vi "CommonVIs_ClassIconSelection.vi"(3 "Offset":T1, 4 "SaveChangesInClassRightAway(True)":bool=TRUE, 5 "IconSelected":refnum<user-event>, 6 "IconsToShow(All)":T2, 7 "Icon":refnum<vi>, 8 "error in (no error)":errorcluster, 9 "Messages(Stop or Empty string will stop this VI)":refnum<user-event>, 10 "IconSelection":refnum<vi>, 11 "LVClassToActOn":refnum<vi>) -> ()   [LabVIEW 2020]
uses:
  <resource>/Framework/Providers/Open_GDS/ClassProviders/Common/CommonVIs/CommonVIs_ClassIconSelection_Action.ctl
  <vilib>/Utility/miscctls.llb/LVPositionTypeDef.ctl
  45c64d35-ac36-4efc-be44-fe8a67d8f3b0.vi
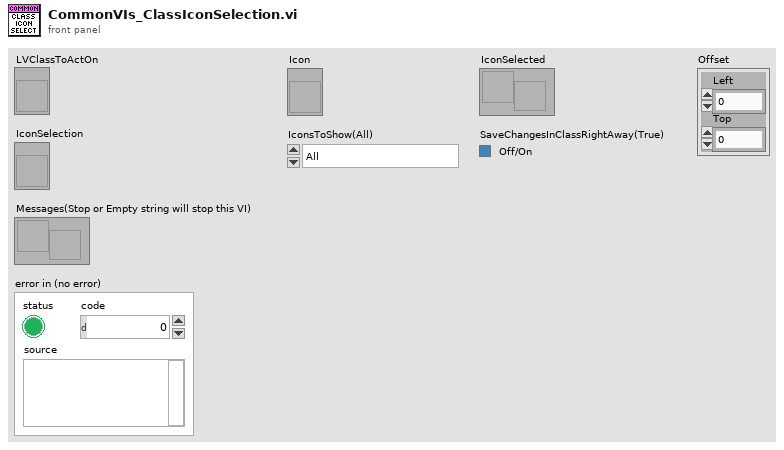
[diagram p1: front panel]
types:
  T1 = typedef "LVPositionTypeDef.ctl" = cluster{"Left":i32, "Top":i32}
  T2 = typedef "CommonVIs_ClassIconSelection_Action.ctl" = enum16{"All", "Non Interface", "Only Interface"}
  T3 = cluster{"SelectedIcon":string, "IconSelection":picture, "CurrentIcon":picture, "Icons":string[][], "MarkedIconSelection":picture, "Timeout":i32}
  T4 = cluster{"Width":i16, "Style":enum32{"Solid", "Dash", "Dot", "DashDot", "DashDotDot"}}
  T5 = cluster{"left":i16, "top":i16, "right":i16, "bottom":i16}
  T6 = typedef "BaseProvider_IniFileSettings.ctl" = cluster{"ClassFolderSuffix":string, "InterfaceFolderSuffix":string, "InterfaceIcon":string}
  T7 = typedef "imagedata.ctl" = cluster{"image type":i32, "image depth":i32, "image":u8[], "mask":u8[], "colors":u32[], "Rectangle":cluster{"left":i16, "top":i16, "right":i16, "bottom":i16}}
  T8 = cluster{"index of element":i32, i32, "index of element":i32, i32}
  T9 = cluster{"IconDimensions":i16, "IconDimensions":i16, "IconDimensions":i16, "IconDimensions":i16}
  T10 = cluster{"index of element":i16, i16, "index of element":i16, i16}
  T11 = typedef "lveventtype.ctl" = enum32{"Null", "Timeout", "Annotation Menu Selection", "Annotation Menu Selection?", "App Instance Close", "App Instance Close?", "Autoscale Range Change", "Bookmark Info Change", "Cell Edit", "Cell Edit?", "Cursor Grab", "Cursor Grab?", "Cursor Menu Selection", "Cursor Menu Selection?", "Cursor Move", "Cursor Release", "Data Change", "Direction Change", "Display State Change", "Drag Ended", "Drag Enter", "Drag Leave", "Drag Over", "Drag Source Update", "Drag Starting", "Drag Starting?", "Drop", "Exec State Change", "Key Down", "Key Down?", "Key Repeat", "Key Repeat?", "Key Up", "Listbox Double Click", "Menu Activation?", "Menu Selection (App)", "Menu Selection? (App)", "Menu Selection (User)", "Mouse Down", "Mouse Down?", "Mouse Enter", "Mouse Leave", "Mouse Move", "Mouse Up", "Mouse Wheel", "NI Security User Change (App)", "Pane Size", "Panel Close", "Panel Close?", "Panel Resize", "Plot Attribute Change", "Scale Range Change", "Shortcut Menu Activation?", "Shortcut Menu Selection (App)", "Shortcut Menu Selection? (App)", "Shortcut Menu Selection (User)", "Tree Double Click", "Tree Drag", "Tree Drag?", "Tree Drop", "Tree Drop?", "Tree Item Close", "Tree Item Close?", "Tree Item Open", "Tree Item Open?", "User Event", "Value Change"}
  T12 = typedef "LVMouseTypeDef.ctl" = cluster{"Mouse Position":cluster{"X":i32, "Y":i32}, "Mouse Modifiers":cluster{"Button Down":bool, "Shift Mod":bool, "Menu Mod":bool, "Option Mod":bool}}
  T13 = cluster{"IconDimensions":i16, "IconDimensions":i16}
  T14 = typedef "Scripting_ConnectorPanePatternType.ctl" = u16
  T15 = typedef "GOOP_WireConfigurationType.ctl" = cluster{"Edge thickness":i32, "Edge color":u32, "Center thickness":i32, "Center pattern":T16, "CenterColor1":u32, "CenterColor2":u32, "Tunnels and terminals colors":u32}
  T16 = typedef "GOOP_WirePattern.ctl" = enum16{"Solid", "Large dash", "Small dash"}
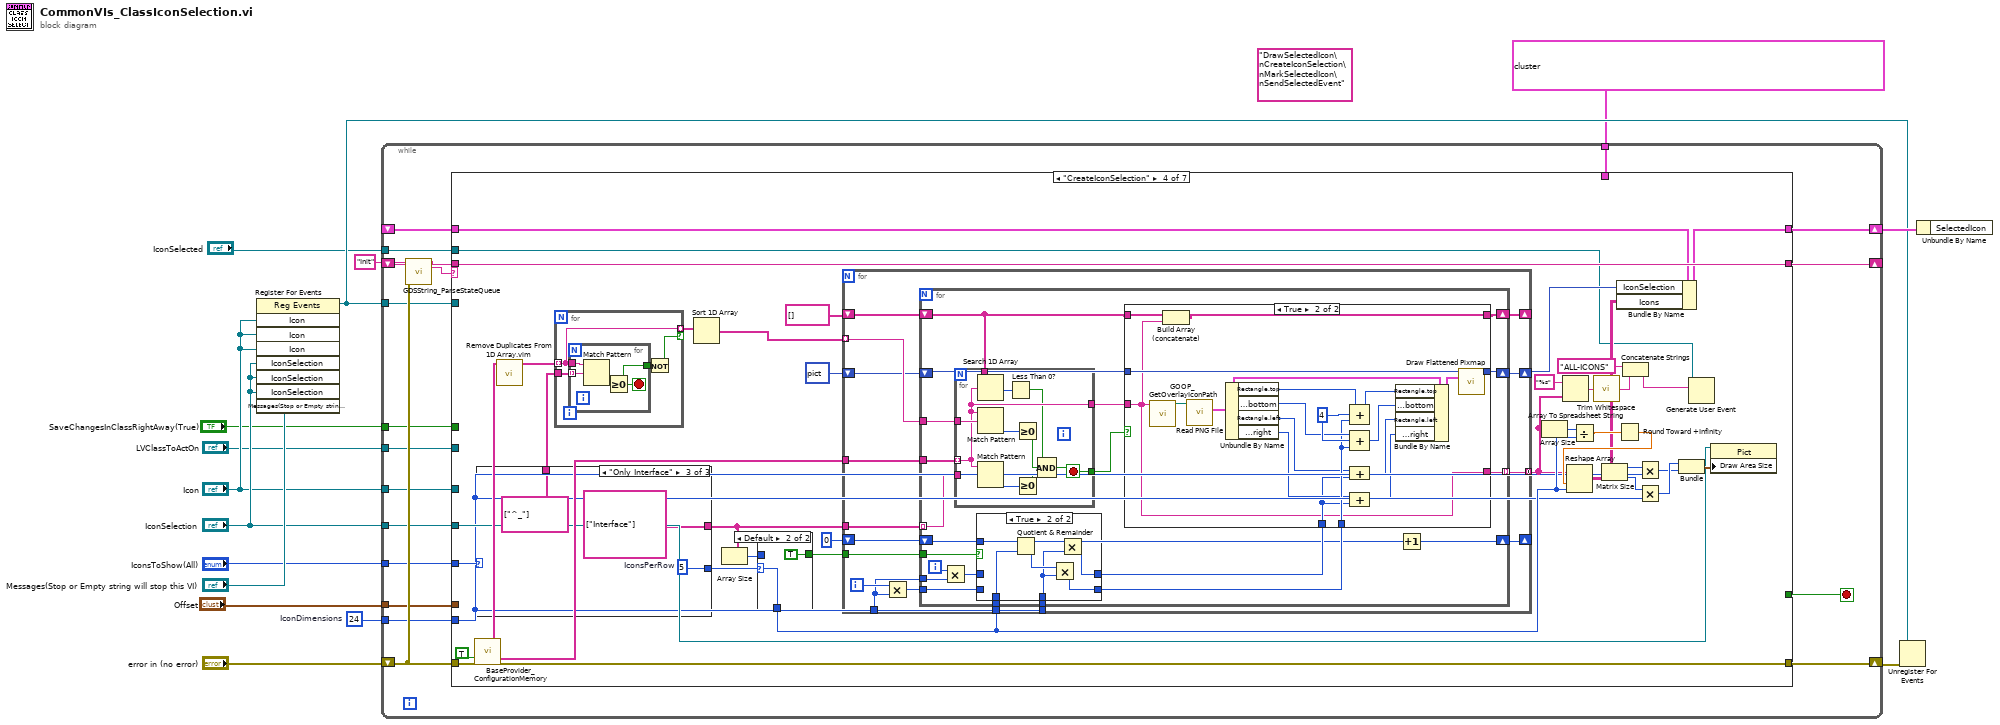
[diagram p0: block diagram]
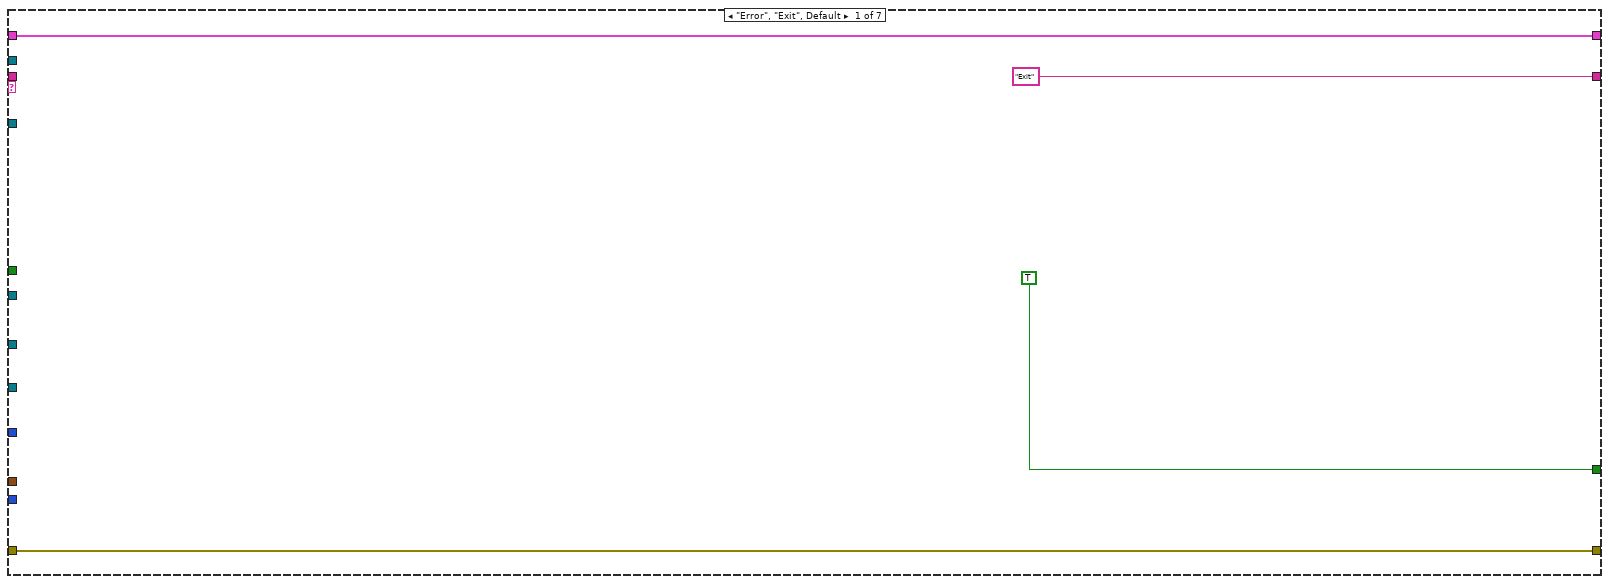
[diagram p2: hidden frame]
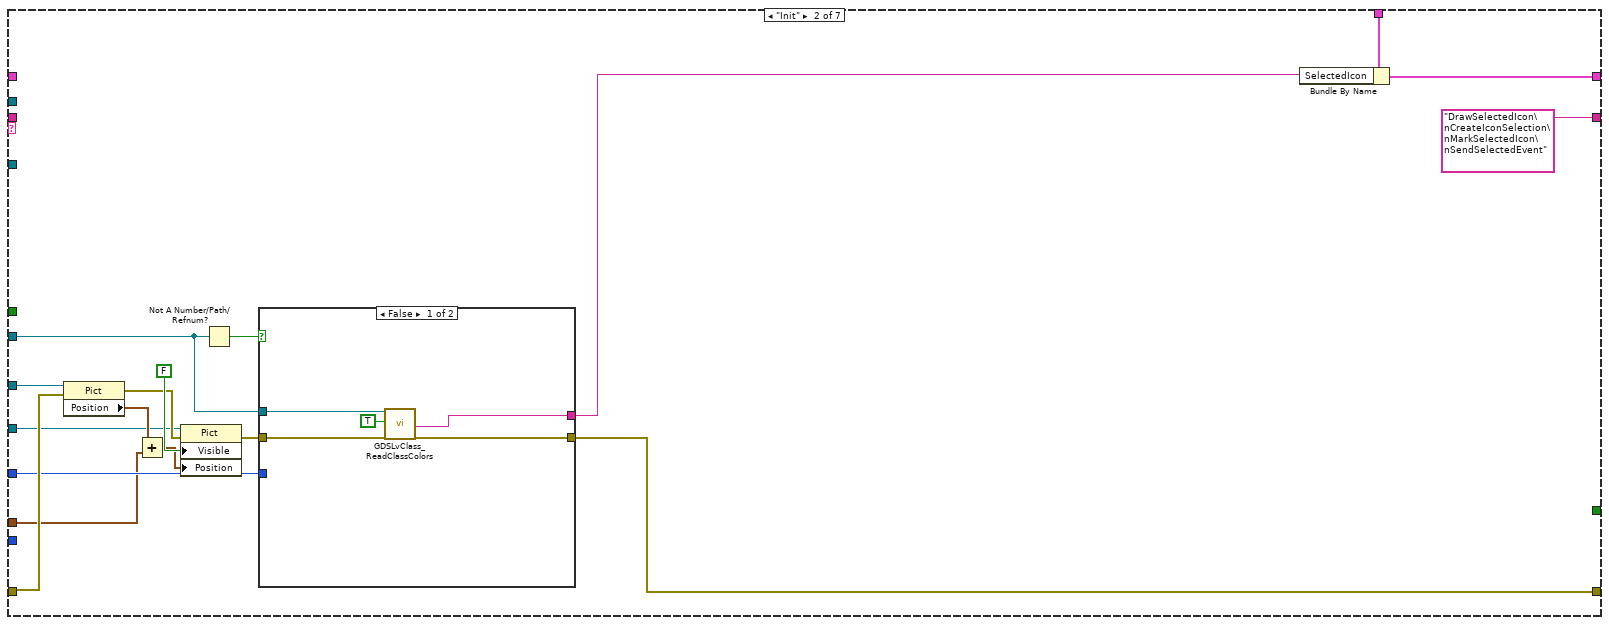
[diagram p3: hidden frame]
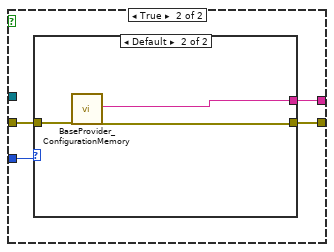
[diagram p4: hidden frame]
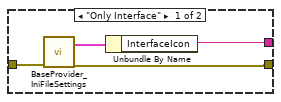
[diagram p5: hidden frame]
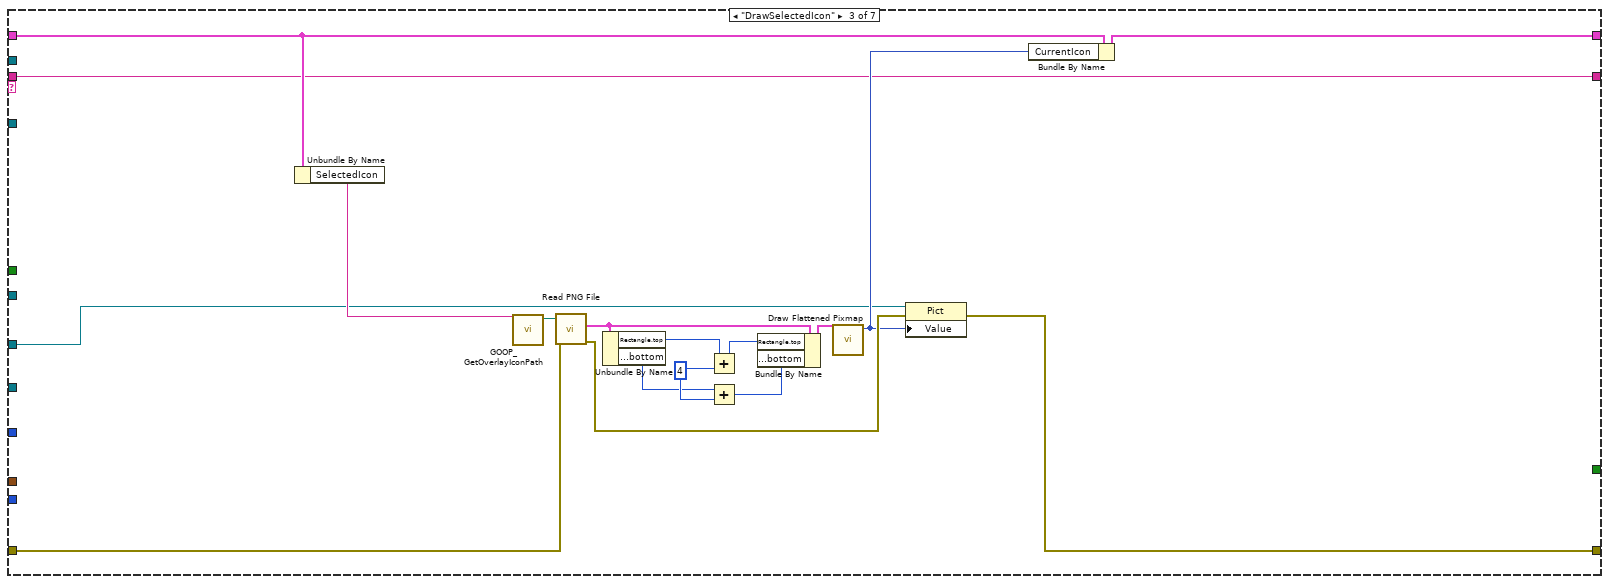
[diagram p6: hidden frame]
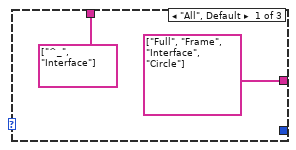
[diagram p8: hidden frame]
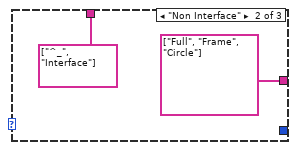
[diagram p9: hidden frame]
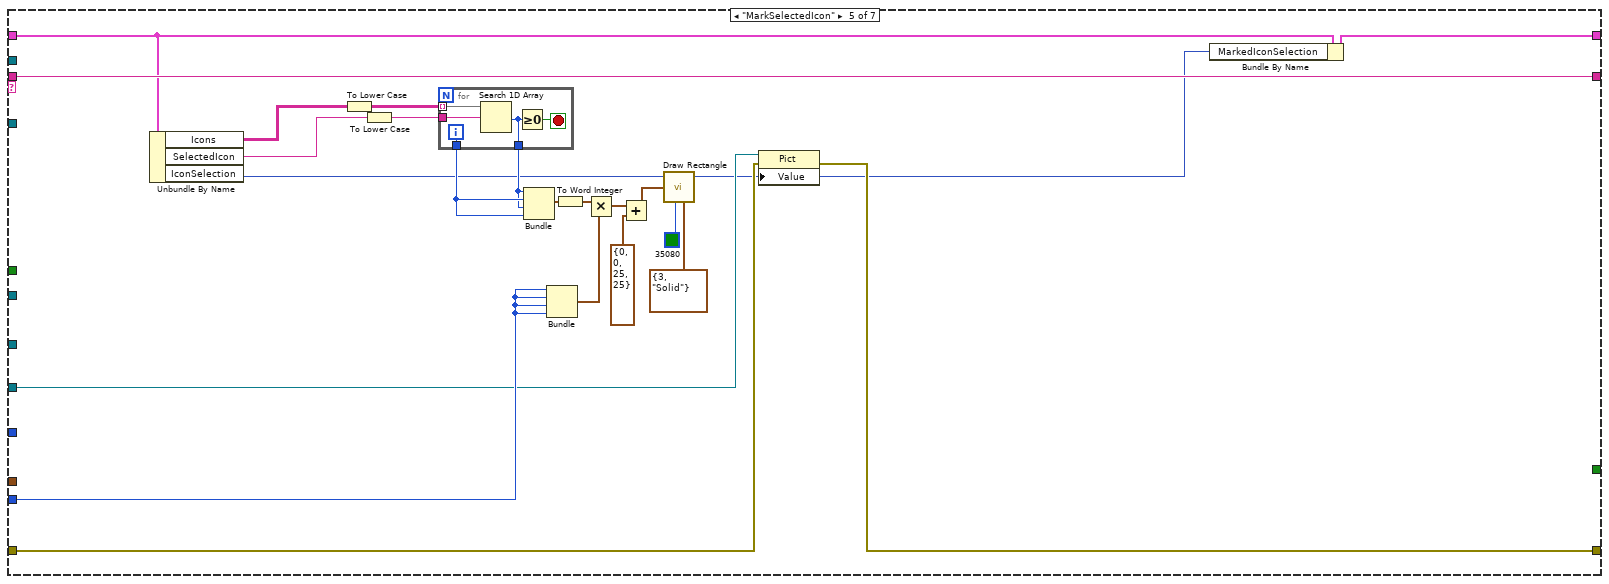
[diagram p12: hidden frame]
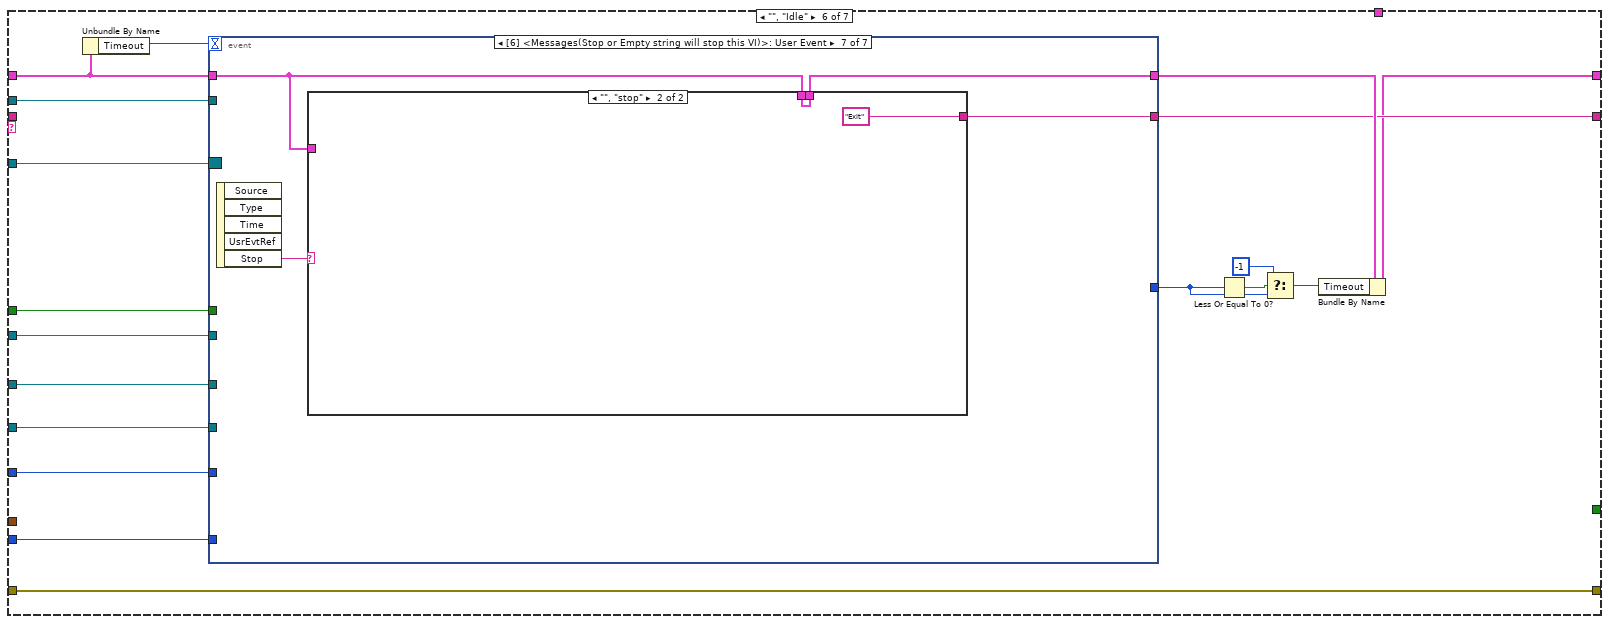
[diagram p13: hidden frame]
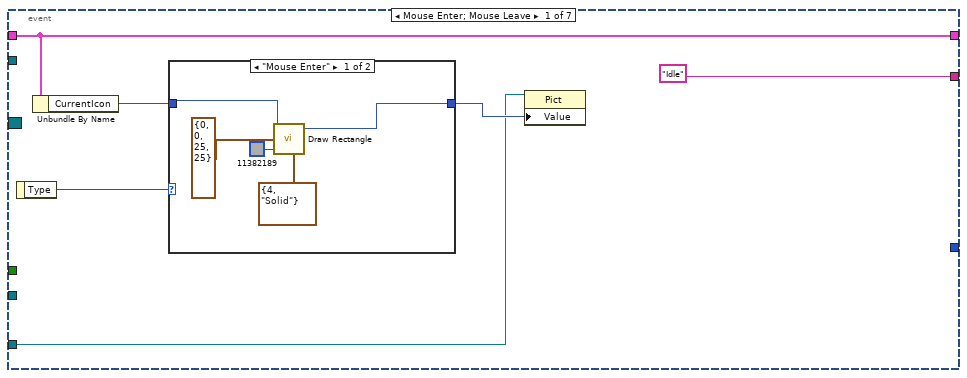
[diagram p14: hidden frame]
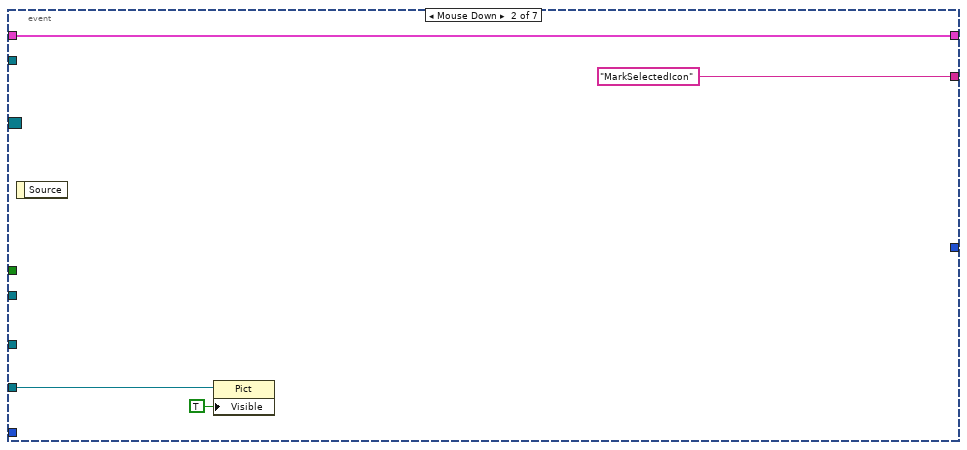
[diagram p16: hidden frame]
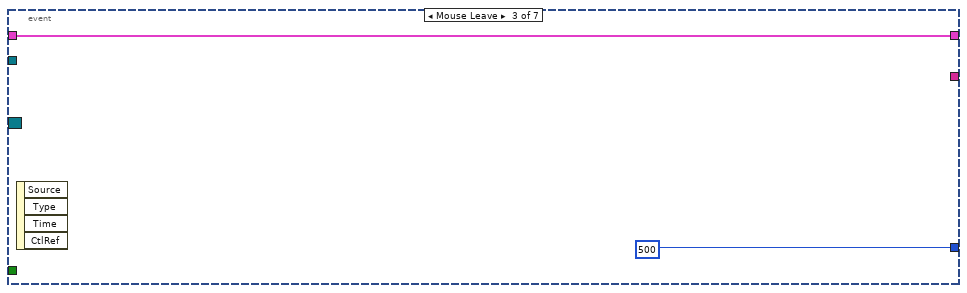
[diagram p17: hidden frame]
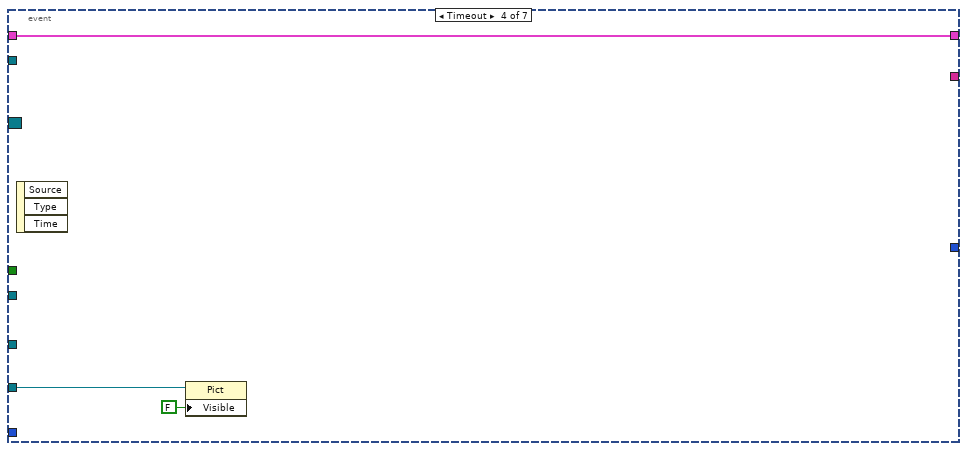
[diagram p18: hidden frame]
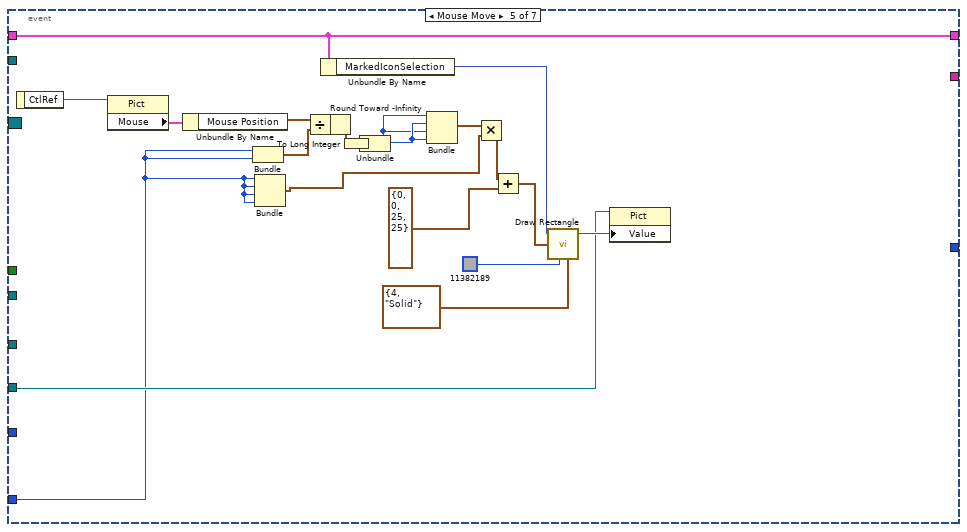
[diagram p19: hidden frame]
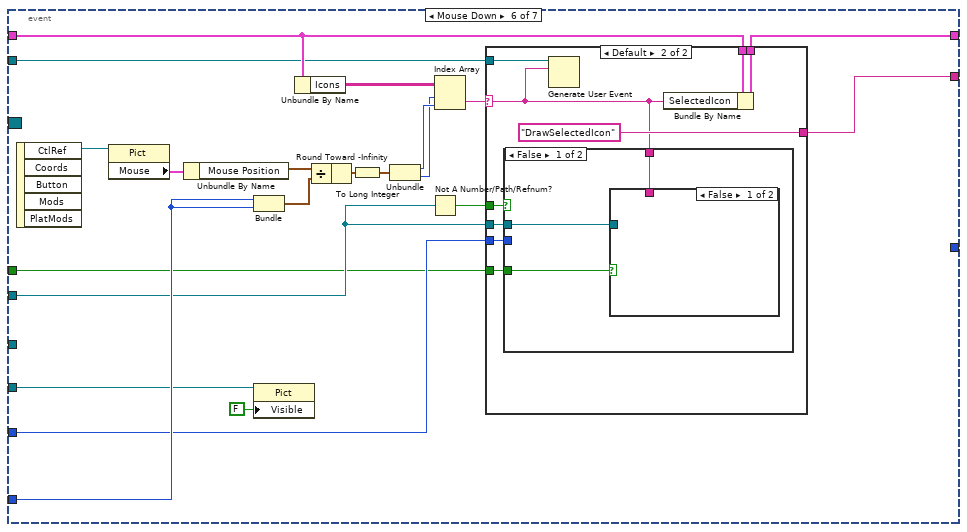
[diagram p20: hidden frame]
diagram:
  (unwired) "DrawSelectedIcon\nCreateIconSelection\nMarkSelectedIcon\nSendSelectedEvent"
  w8 = i16 24  # IconDimensions
  n1 = register-events("Icon", "Icon", "Icon", "IconSelection", "IconSelection", "IconSelection", "Messages(Stop or Empty string will stop this VI)") -> (reference out=w12:refnum<event-registration>)  [unwired: 2 in, 1 out]
  n2 = while {
    shift-right: [w30] -> w11
    shift-left: "error in (no error)" -> [w33]
    shift-right: [w29] -> _
    shift-left: "Init" -> [w34]
    tunnel: "IconSelection" -> [w32]
    tunnel: "Icon" -> [w31]
    tunnel: w8 -> [w25]
    tunnel: T3 {"SelectedIcon"="", "IconSelection"=bytes[0], "CurrentIcon"=bytes[0], "Icons"=[], "MarkedIconSelection"=bytes[0], "Timeout"=-1} -> [w24]
    shift-right: [w23] -> w14
    shift-left: _ -> [w22]
    tunnel: w12 -> [w21]
    tunnel: "IconsToShow(All)" -> [w20]
    tunnel: "LVClassToActOn" -> [w19]
    tunnel: "IconSelected" -> [w18]
    tunnel: "SaveChangesInClassRightAway(True)" -> [w17]
    tunnel: "Offset" -> [w16]
    stop <- w28 stop-if-true
    n3 = call <resource>:"GDSString_ParseStateQueue.vi"("State Queue"=w34, "Error In (no error)"=w33) -> ("Remaining States"=w27:string, "Current State"=w26:string)  [unwired: 9 in, 3 out]
    n4 = case shown="\"CreateIconSelection\"" w26 {
      tunnel: w33 -> [w38 w53 w76 w126 w230 w270 w389]
      tunnel: w32 -> [_ w47 _ w111 w232 w266 _]
      tunnel: w31 -> [_ w48 w72 _ _ w257 _]
      tunnel: [w38 w46 w77 w127 w231 w270 w389] -> w30
      tunnel: ["Exit" "DrawSelectedIcon\nCreateIconSelection\nMarkSelectedIcon\nSendSelectedEvent" w73 w128 w247 w267 w388] -> w29
      tunnel: [TRUE _ _ _ _ _ _] -> w28
      tunnel: w27 -> [_ _ w73 w128 w247 _ w388]
      tunnel: w25 -> [_ _ _ w98 w234 w265 _]
      tunnel: w24 -> [_ w50 _ _ _ _ _]
      tunnel: [w35 w49 w75 w110 w229 w264 w386] -> w23
      tunnel: w22 -> [w35 _ w79 w117 w246 w259 w386]
      tunnel: w21 -> [_ _ _ _ _ w269 _]
      tunnel: w20 -> [_ w44 _ w108 _ w256 _]
      tunnel: w19 -> [_ w42 _ _ _ w255 _]
      tunnel: w18 -> [_ _ _ w94 _ w254 w387]
      tunnel: w17 -> [_ _ _ _ _ w253 _]
      tunnel: w16 -> [_ w39 _ _ _ _ _]
      frame "Error", "Exit", Default {
      }
      frame "Init" {
        n5 = property class="Pict"(reference=w48, error in=w53) -> (error out=w52:errorcluster, "Position"=w55:T1)  [unwired: 1 out]
        n6 = Add(x=w55, y=w39) -> (x+y=w40:T1)
        n7 = property class="Pict"(reference=w47, error in=w52, "Visible"=FALSE, "Position"=w40) -> (error out=w51:errorcluster)  [unwired: 1 out]
        n8 = Not A Number/Path/Refnum?(number/path/refnum=w42) -> (NaN/Path/Refnum?=w43:bool)
        n9 = case shown="False" w43 {
          tunnel: w51 -> [w60 w64]
          tunnel: [w58 w63] -> w46
          tunnel: [w57 w62] -> w45
          tunnel: w44 -> [_ w61]
          tunnel: w42 -> [w59 _]
          frame False {
            n10 = call <resource>:"GDSLvClass_ReadClassColors.vi"("Library Refnum"=w59, "OnlyReadClassItemIcon(False)"=TRUE, "error in (no error)"=w60) -> ("ClassItemIconName(NoExtension)"=w57:string, "error out"=w58:errorcluster)  [unwired: 11 in, 4 out]
          }
          frame True {
            n11 = case shown="Default" w61 {
              tunnel: w64 -> [w68 w71]
              tunnel: [w67 w70] -> w63
              tunnel: [w65 w69] -> w62
              frame "Only Interface" {
                n12 = call <resource>:"BaseProvider_IniFileSettings.vi"("error in (no error)"=w68) -> ("IniFileSettings"=w66:T6, "error out"=w67:errorcluster)  [unwired: 17 in]
                n13 = Unbundle By Name(w66) -> ("InterfaceIcon"=w65:string)
              }
              frame Default {
                n14 = call <resource>:"BaseProvider_ConfigurationMemory.vi"("error in (no error)"=w71) -> ("IconOut"=w69:string, "error out"=w70:errorcluster)  [unwired: 12 in, 5 out]
              }
            }
          }
        }
        n15 = Bundle By Name(cluster=w50, "SelectedIcon"=w45) -> (w49:T3)
      }
      frame "DrawSelectedIcon" {
        w88 = i16 4 ("y")
        n16 = Unbundle By Name(w79) -> ("SelectedIcon"=w78:string)
        n17 = call <resource>:"GOOP_GetOverlayIconPath.vi"("IconName(NoPngExtension)"=w78) -> ("IconPath"=w81:path)  [unwired: 10 in]
        n18 = call <vilib>:"Read PNG File.vi"("error in (no error)"=w76, "path to PNG file"=w81) -> ("error out"=w80:errorcluster, "image data"=w83:T7)  [unwired: 7 in, 1 out]
        n19 = Unbundle By Name(w83) -> ("Rectangle.top"=w84:i16, "Rectangle.bottom"=w85:i16)
        n20 = Add(x=w84, y=w88) -> (x+y=w86:i16)
        n21 = Add(x=w85, y=w88) -> (x+y=w87:i16)
        n22 = Bundle By Name(cluster=w83, "Rectangle.top"=w86, "Rectangle.bottom"=w87) -> (w82:T7)
        n23 = call <vilib>:"Draw Flattened Pixmap.vi"("image data"=w82) -> ("new picture"=w74:picture)  [unwired: 8 in]
        n24 = property class="Pict"(reference=w72, error in=w80, "Value"=w74) -> (error out=w77:errorcluster)  [unwired: 1 out]
        n25 = Bundle By Name(cluster=w79, "CurrentIcon"=w74) -> (w75:T3)
      }
      frame "CreateIconSelection" {
        n26 = call <resource>:"BaseProvider_ConfigurationMemory.vi"("Filter_Icons"=TRUE, "error in (no error)"=w126) -> ("ClassItemIconGroup"=w122:string[], "ClassItemIconNames"=w118:string[], "error out"=w127:errorcluster)  [unwired: 11 in, 4 out]
        n27 = case shown="\"Only Interface\"" w108 {
          tunnel: [string[] ["^_", "Interface"] ("element") string[] ["^_", "Interface"] ("element") string[] ["^_"] ("element")] -> w124
          tunnel: [string[] ["Full", "Frame", "Interface", "Circle"] ("element") string[] ["Full", "Frame", "Circle"] ("element") string[] ["Interface"] ("element")] -> w107
          tunnel: [_ _ w136] -> w106
          frame "All", Default {
          }
          frame "Non Interface" {
          }
          frame "Only Interface" {
            w136 = i16 5  # IconsPerRow
          }
        }
        n28 = call "Remove Duplicates From 1D Array.vim"("array"=w122) -> ("array with duplicates removed"=w123:string[])  [unwired: 10 in]
        n29 = for {
          tunnel: w123 -> [w218] mode=indexing
          tunnel: w124 -> [w220]
          tunnel: [w218] -> w125 mode=indexing if=w217
          n30 = for {
            tunnel: w218 -> [w224]
            tunnel: w220 -> [w223] mode=indexing
            tunnel: [w221] -> w219
            stop <- w221 stop-if-true
            n31 = Match Pattern(string=w224, regular expression=w223) -> (offset past match=w222:i32)  [unwired: 1 in, 3 out]
            n32 = Greater Or Equal To 0?(x=w222) -> (x >= 0?=w221:bool)
          }
          n33 = Not(x=w219) -> (.not. x?=w217:bool)
        }
        n34 = Sort 1D Array(array=w125) -> (sorted array=w119:string[])
        n35 = Array Size(array=w107) -> (size(s)=w105:i32)
        n36 = case shown="Default" w106 {
          selector: w106 -> [_ w131]
          tunnel: w105 -> [w129 _]
          tunnel: [w129 w131] -> w99
          tunnel: [_ TRUE] -> w100
          frame 0 {
          }
          frame Default {
          }
        }
        n37 = for {
          tunnel: w119 -> [w152] mode=indexing
          tunnel: w107 -> [w153]
          tunnel: [w151] -> w96 mode=concatenating
          shift-right: [w149] -> w109
          shift-left: picture data[5B] ("new picture") -> [w150]
          shift-right: [w145] -> _
          shift-left: string[] [] -> [w154]
          tunnel: w118 -> [w146]
          tunnel: w98 -> [w144]
          shift-right: [w139] -> _
          shift-left: i16 0 ("y") -> [w143]
          tunnel: w100 -> [w142]
          tunnel: w99 -> [w141]
          tunnel: w98 -> [w140]
          i -> [w148]
          n38 = Multiply(x=w148, y=w144) -> (x*y=w147:i32)
          n39 = for {
            tunnel: w153 -> [w174] mode=indexing
            tunnel: w152 -> [w175]
            tunnel: [w164] -> w151 mode=indexing
            shift-right: [w172] -> w149
            shift-left: w150 -> [w173]
            tunnel: w147 -> [w162]
            tunnel: w144 -> [w168]
            shift-right: [w166] -> w145
            shift-left: w154 -> [w165]
            tunnel: w146 -> [w167]
            shift-right: [w155] -> w139
            shift-left: w143 -> [w156]
            tunnel: w142 -> [w161]
            tunnel: w141 -> [w160]
            tunnel: w140 -> [w159]
            i -> [w169]
            n40 = Multiply(x=w169, y=w168) -> (x*y=w163:i32)
            n41 = for {
              tunnel: w167 -> [w187] mode=indexing
              tunnel: w175 -> [w195]
              tunnel: w174 -> [w193]
              tunnel: [w189] -> w171
              tunnel: [w187] -> w170
              tunnel: w165 -> [w188]
              stop <- w189 stop-if-true
              n42 = Search 1D Array(1D array=w188, element=w187) -> (index of element=w186:i32)  [unwired: 1 in]
              n43 = Match Pattern(string=w187, regular expression=w195) -> (offset past match=w194:i32)  [unwired: 1 in, 3 out]
              n44 = Match Pattern(string=w187, regular expression=w193) -> (offset past match=w192:i32)  [unwired: 1 in, 3 out]
              n45 = Less Than 0?(x=w186) -> (x < 0?=w185:bool)
              n46 = Greater Or Equal To 0?(x=w194) -> (x >= 0?=w191:bool)
              n47 = Greater Or Equal To 0?(x=w192) -> (x >= 0?=w190:bool)
              n48 = Compound Arithmetic op=AND(w185, w191, w190) -> (w189:bool)
            }
            n49 = case shown="True" w161 {
              tunnel: w163 -> [w177 _]
              tunnel: w162 -> [w176 _]
              tunnel: w156 -> [_ w184]
              tunnel: w160 -> [_ w183]
              tunnel: w159 -> [_ w179]
              tunnel: [w177 w181] -> w158
              tunnel: [w176 w178] -> w157
              frame False {
              }
              frame True {
                n50 = Quotient & Remainder(x=w184, y=w183) -> (x-y*floor(x/y)=w182:i32, floor(x/y)=w180:i32)
                n51 = Multiply(x=w180, y=w179) -> (x*y=w178:i32)
                n52 = Multiply(x=w182, y=w179) -> (x*y=w181:i32)
              }
            }
            n53 = case shown="True" w171 {
              tunnel: w173 -> [w197 w209]
              tunnel: [w197 w208] -> w172
              tunnel: w170 -> [_ w198]
              tunnel: w157 -> [_ w206]
              tunnel: w158 -> [_ w201]
              tunnel: w165 -> [w196 w200]
              tunnel: [w196 w199] -> w166
              tunnel: [_ w198] -> w164
              frame False {
              }
              frame True {
                w215 = i16 4 ("y")
                n54 = call <resource>:"GOOP_GetOverlayIconPath.vi"("IconName(NoPngExtension)"=w198) -> ("IconPath"=w216:path)  [unwired: 10 in]
                n55 = Build Array (concatenate)(w200, w198) -> (w199:string[])
                n56 = call <vilib>:"Read PNG File.vi"("path to PNG file"=w216) -> ("image data"=w207:T7)  [unwired: 8 in, 2 out]
                n57 = Unbundle By Name(w207) -> ("Rectangle.top"=w211:i16, "Rectangle.bottom"=w212:i16, "Rectangle.left"=w205:i16, "Rectangle.right"=w204:i16)
                n58 = Compound Arithmetic op=ADD(w211, w215, w206) -> (w213:i32)
                n59 = Compound Arithmetic op=ADD(w212, w215, w206) -> (w214:i32)
                n60 = Compound Arithmetic op=ADD(w205, w201) -> (w203:i32)
                n61 = Compound Arithmetic op=ADD(w204, w201) -> (w202:i32)
                n62 = Bundle By Name(cluster=w207, "Rectangle.top"=w213, "Rectangle.bottom"=w214, "Rectangle.left"=w203, "Rectangle.right"=w202) -> (w210:T7)
                n63 = call <vilib>:"Draw Flattened Pixmap.vi"("image data"=w210, "picture"=w209) -> ("new picture"=w208:picture)  [unwired: 7 in]
              }
            }
            n64 = Increment(x=w156) -> (x+1=w155:i16)
          }
        }
        n65 = Array Size(array=w96) -> (size(s)=w104:i32)
        n66 = Array To Spreadsheet String(array=w96, 3:"%s" ("format string")) -> (spreadsheet string=w93:string)  [unwired: 1 in]
        n67 = Divide(x=w104, y=w99) -> (x/y=w103:dbl)
        n68 = call <vilib>:"Trim Whitespace.vi"("string"=w93) -> ("trimmed string"=w90:string)  [unwired: 1 in]
        n69 = Round Toward +Infinity(x=w103) -> (ceil(x): smallest int >= x=w102:dbl)
        n70 = Reshape Array(w96, w102, w99) -> (w97:string[][])
        n71 = Matrix Size(0:w97) -> (1:w113:i32, 2:w114:i32)
        n72 = Bundle By Name(cluster=w117, "IconSelection"=w109, "Icons"=w97) -> (w110:T3)
        n73 = Concatenate Strings("ALL-ICONS" ("string"), w90) -> (w92:string)
        n74 = Multiply(x=w113, y=w98) -> (x*y=w115:i32)
        n75 = Multiply(x=w114, y=w98) -> (x*y=w116:i32)
        n76 = Bundle(w116, w115) -> (w112:cluster{i32, i32})  [unwired: 1 in]
        n77 = Generate User Event(user event=w94, event data cluster=w92) -> ()  [unwired: 2 in, 2 out]
        n78 = property on="Property Node" class="Pict"(reference=w111, "Draw Area Size"=w112) -> ()  [unwired: 1 in, 2 out]
      }
      frame "MarkSelectedIcon" {
        n79 = Unbundle By Name(w246) -> ("Icons"=w235:string[][], "SelectedIcon"=w225:string, "IconSelection"=w236:picture)
        n80 = To Lower Case(string=w235) -> (all lower case string=w226:string[][])
        n81 = To Lower Case(string=w225) -> (all lower case string=w227:string)
        n82 = for {
          tunnel: w226 -> [w252] mode=indexing
          tunnel: w227 -> [w251]
          tunnel: [w249] -> w240
          tunnel: [w248] -> w239
          i -> [w249]
          stop <- w250 stop-if-true
          n83 = Search 1D Array(1D array=w252, element=w251) -> (index of element=w248:i32)  [unwired: 1 in]
          n84 = Greater Or Equal To 0?(x=w248) -> (x >= 0?=w250:bool)
        }
        n85 = Bundle("index of element"=w239, w240, "index of element"=w239, w240) -> (w238:T8)  [unwired: 1 in]
        n86 = Bundle("IconDimensions"=w234, "IconDimensions"=w234, "IconDimensions"=w234, "IconDimensions"=w234) -> (w241:T9)  [unwired: 1 in]
        n87 = To Word Integer(number=w238) -> (16bit integer=w233:T10)
        n88 = Multiply(x=w233, y=w241) -> (x*y=w242:cluster{i16, i16, i16, i16})
        n89 = Add(x=w242, y=T5 {"left"=0, "top"=0, "right"=25, "bottom"=25} ("rect")) -> (x+y=w244:cluster{i16, i16, i16, i16})
        n90 = call <vilib>:"Draw Rectangle.vi"("picture"=w236, "rect"=w244, "color(black)"=u32 35080, "pen"=T4 {"Width"=3, "Style"=enum."Solid"}) -> ("new picture"=w228:picture)  [unwired: 5 in]
        n91 = property class="Pict"(reference=w232, error in=w230, "Value"=w228) -> (error out=w231:errorcluster)  [unwired: 1 out]
        n92 = Bundle By Name(cluster=w246, "MarkedIconSelection"=w228) -> (w229:T3)
      }
      frame "", "Idle" {
        n93 = Unbundle By Name(w259) -> ("Timeout"=w258:i32)
        n94 = event shown="[6] <Messages(Stop or Empty string will stop this VI)>: User Event" {
          selector: w269 -> [_ _ _ _ _ _ _]
          dyn-events: _ -> [_ _ _ _ _ _ _]
          timeout: w258 -> [_ _ _ _ _ _ _]
          tunnel: w259 -> [w274 w284 w288 w291 w297 w326 w363]
          tunnel: [w274 w284 w288 w291 w297 w324 w364] -> w268
          tunnel: ["Idle" "MarkSelectedIcon" _ _ _ w322 w365] -> w267
          tunnel: w266 -> [_ w286 _ w289 w294 w320 _]
          tunnel: w265 -> [_ _ _ _ w293 w327 _]
          tunnel: [_ _ 500 ("500") _ _ _ _] -> w261
          tunnel: w257 -> [w271 _ _ _ _ _ _]
          tunnel: w256 -> [_ _ _ _ _ w317 _]
          tunnel: w255 -> [_ _ _ _ _ w315 _]
          tunnel: w254 -> [_ _ _ _ _ w314 _]
          tunnel: w253 -> [_ _ _ _ _ w313 _]
          event Mouse Enter; Mouse Leave {
            n95 = event-data() -> ("Type"=w276:T11)  [unwired: 1 in]
            n96 = Unbundle By Name(w274) -> ("CurrentIcon"=w273:picture)
            n97 = case shown="\"Mouse Enter\"" w276 {
              tunnel: [w279 w282] -> w275
              tunnel: w273 -> [w278 w282]
              frame "Mouse Enter" {
                n98 = call <vilib>:"Draw Rectangle.vi"("picture"=w278, "rect"=T5 {"left"=0, "top"=0, "right"=25, "bottom"=25}, "color(black)"=u32 11382189, "pen"=T4 {"Width"=4, "Style"=enum."Solid"}) -> ("new picture"=w279:picture)  [unwired: 5 in]
              }
              frame "Mouse Leave", Default {
              }
            }
            n99 = property class="Pict"(reference=w271, "Value"=w275) -> ()  [unwired: 1 in, 2 out]
          }
          event Mouse Down {
            n100 = event-data() -> ()  [unwired: 1 in, 1 out]
            n101 = property class="Pict"(reference=w286, "Visible"=TRUE) -> ()  [unwired: 1 in, 2 out]
          }
          event Mouse Leave {
            n102 = event-data() -> ()  [unwired: 1 in, 4 out]
          }
          event Timeout {
            n103 = event-data() -> ()  [unwired: 1 in, 3 out]
            n104 = property class="Pict"(reference=w289, "Visible"=FALSE) -> ()  [unwired: 1 in, 2 out]
          }
          event Mouse Move {
            n105 = event-data() -> ("CtlRef"=w299:refnum<vi>)  [unwired: 1 in]
            n106 = property on="Property Node" class="Pict"(reference=w299) -> ("Mouse"=w300:T12)  [unwired: 1 in, 2 out]
            n107 = Unbundle By Name(w300) -> ("Mouse Position"=w301:cluster{"X":i32, "Y":i32})
            n108 = Bundle("IconDimensions"=w293, "IconDimensions"=w293) -> (w298:T13)  [unwired: 1 in]
            n109 = Bundle("IconDimensions"=w293, "IconDimensions"=w293, "IconDimensions"=w293, "IconDimensions"=w293) -> (w292:T9)  [unwired: 1 in]
            n110 = Divide(x=w301, y=w298) -> (x/y=w302:cluster{dbl, dbl})
            n111 = Unbundle By Name(w297) -> ("MarkedIconSelection"=w296:picture)
            n112 = Round Toward -Infinity(1:w302) -> (0:w303:cluster{dbl, dbl})
            n113 = To Long Integer(number=w303) -> (32bit integer=w308:cluster{i32, i32})
            n114 = Unbundle(w308) -> (w306:i32, w307:i32)
            n115 = Bundle(w306, w307, w306, w307) -> (w309:cluster{i32, i32, i32, i32})  [unwired: 1 in]
            n116 = Multiply(x=w309, y=w292) -> (x*y=w311:cluster{i32, i32, i32, i32})
            n117 = Add(x=w311, y=T5 {"left"=0, "top"=0, "right"=25, "bottom"=25} ("rect")) -> (x+y=w312:cluster{i32, i32, i32, i32})
            n118 = call <vilib>:"Draw Rectangle.vi"("picture"=w296, "rect"=w312, "color(black)"=u32 11382189, "pen"=T4 {"Width"=4, "Style"=enum."Solid"}) -> ("new picture"=w295:picture)  [unwired: 5 in]
            n119 = property class="Pict"(reference=w294, "Value"=w295) -> ()  [unwired: 1 in, 2 out]
          }
          event Mouse Down {
            n120 = event-data() -> ("CtlRef"=w328:refnum<vi>)  [unwired: 1 in, 4 out]
            n121 = property on="Property Node" class="Pict"(reference=w328) -> ("Mouse"=w330:T12)  [unwired: 1 in, 2 out]
            n122 = Unbundle By Name(w330) -> ("Mouse Position"=w331:cluster{"X":i32, "Y":i32})
            n123 = Bundle("IconDimensions"=w327, "IconDimensions"=w327) -> (w329:T13)  [unwired: 1 in]
            n124 = property class="Pict"(reference=w320, "Visible"=FALSE) -> ()  [unwired: 1 in, 2 out]
            n125 = Unbundle By Name(w326) -> ("Icons"=w325:string[][])
            n126 = Divide(x=w331, y=w329) -> (x/y=w332:cluster{dbl, dbl})
            n127 = Round Toward -Infinity(1:w332) -> (0:w333:cluster{dbl, dbl})
            n128 = To Long Integer(number=w333) -> (32bit integer=w334:cluster{i32, i32})
            n129 = Unbundle(w334) -> (w319:i32, w318:i32)
            n130 = Not A Number/Path/Refnum?(number/path/refnum=w315) -> (NaN/Path/Refnum?=w316:bool)
            n131 = Index Array(array=w325, index (row)=w318, index (col)=w319) -> (element=w323:string)
            n132 = case shown="Default" w323 {
              selector: w323 -> [_ w338]
              tunnel: w326 -> [w335 w344]
              tunnel: [w335 w343] -> w324
              tunnel: [_ "DrawSelectedIcon"] -> w322
              tunnel: w317 -> [_ w341]
              tunnel: w316 -> [_ w340]
              tunnel: w315 -> [_ w339]
              tunnel: w314 -> [_ w337]
              tunnel: w313 -> [_ w336]
              frame "" {
              }
              frame Default {
                n133 = case shown="False" w340 {
                  tunnel: w338 -> [w346 w353]
                  tunnel: w341 -> [_ w352]
                  tunnel: w339 -> [w347 _]
                  tunnel: w336 -> [w345 _]
                  frame False {
                    n134 = case shown="False" w345 {
                      tunnel: w347 -> [_ w351]
                      tunnel: w346 -> [_ w350]
                      frame False {
                      }
                      frame True {
                        n135 = call <resource>:"GDSLvClass_StoreClassItemIcon.vi"("Library Refnum"=w351, "ClassItemIconName"=w350) -> ("Library Refnum"=w349:refnum<vi>, "error out"=w348:errorcluster)  [unwired: 16 in]
                        n136 = invoke class="Library" method="Save"(reference=w349, error in=w348) -> ()  [unwired: 2 in, 4 out]
                      }
                    }
                  }
                  frame True {
                    n137 = case shown="\"Only Interface\"" w352 {
                      tunnel: w353 -> [w354 w360]
                      frame "Only Interface" {
                        n138 = call <resource>:"BaseProvider_IniFileSettings.vi"() -> ("IniFileSettings"=w356:T6, "error out"=w358:errorcluster)  [unwired: 18 in]
                        n139 = Bundle By Name(cluster=w356, "InterfaceIcon"=w354) -> (w355:T6)
                        n140 = call <resource>:"BaseProvider_IniFileSettings.vi"("IniFileSettings"=w355, "error in (no error)"=w358, "Action"=enum16{"Read", "Load", "Save"}."Save") -> ()  [unwired: 15 in, 2 out]
                      }
                      frame Default {
                        n141 = call <resource>:"BaseProvider_ConfigurationMemory.vi"() -> ("PatternOut"=w362:T14, "WireConfigurationOut"=w361:T15)  [unwired: 13 in, 5 out]
                        n142 = call <resource>:"BaseProvider_ConfigurationMemory.vi"("WireConfiguration"=w361, "Icon"=w360, "Action"=enum16{"Read", "Load", "Save", "Set"}."Save", "PatternIn"=w362) -> ()  [unwired: 9 in, 7 out]
                      }
                    }
                  }
                }
                n143 = Generate User Event(user event=w337, event data cluster=w338) -> ()  [unwired: 2 in, 2 out]
                n144 = Bundle By Name(cluster=w344, "SelectedIcon"=w338) -> (w343:T3)
              }
            }
          }
          event User Event {
            n145 = event-data() -> ("Stop"=w366:string)  [unwired: 1 in, 4 out]
            n146 = case shown="\"\", \"stop\"" w366 {
              selector: w366 -> [w370 _]
              tunnel: ["DrawSelectedIcon\nMarkSelectedIcon" "Exit"] -> w365
              tunnel: w363 -> [w377 w383]
              tunnel: [w376 w383] -> w364
              tunnel: w363 -> [w375 _]
              frame Default {
                n147 = Unbundle By Name(w375) -> ("Icons"=w374:string[][], "SelectedIcon"=w369:string)
                n148 = To Lower Case(string=w370) -> (all lower case string=w372:string)
                n149 = To Lower Case(string=w374) -> (all lower case string=w373:string[][])
                n150 = for {
                  tunnel: w373 -> [w382] mode=indexing
                  tunnel: w372 -> [w381]
                  tunnel: [w380] -> _
                  tunnel: [w378] -> w371
                  i -> [w380]
                  stop <- w378 stop-if-true
                  n151 = Search 1D Array(1D array=w382, element=w381) -> (index of element=w379:i32)  [unwired: 1 in]
                  n152 = Greater Or Equal To 0?(x=w379) -> (x >= 0?=w378:bool)
                }
                n153 = Select(t=w370, s=w371, f=w369) -> (s? t:f=w368:string)
                n154 = Bundle By Name(cluster=w377, "SelectedIcon"=w368) -> (w376:T3)
              }
              frame "", "stop" {
              }
            }
          }
        }
        n155 = Less Or Equal To 0?(x=w261) -> (x <= 0?=w263:bool)
        n156 = Select(t=-1, s=w263, f=w261) -> (s? t:f=w262:i32)
        n157 = Bundle By Name(cluster=w268, "Timeout"=w262) -> (w264:T3)
      }
      frame "SendSelectedEvent" {
        n158 = Unbundle By Name(w386) -> ("SelectedIcon"=w385:string)
        n159 = Generate User Event(user event=w387, event data cluster=w385) -> ()  [unwired: 2 in, 2 out]
      }
    }
  }
  n160 = Unregister For Events(event registration refnum=w12, error in=w11) -> ()  [unwired: 1 out]
  n161 = Unbundle By Name(w14) -> ()  [unwired: 1 out]
